vi "OpenExistingDataLogFile.vi"(6 "Chunk Read size, bytes":i32, 8 "error in (no error)":errorcluster, 9 "ExistingFilePath":path, 11 "ExistingFileMgr in":refnum<class "ExistingFileMgr.lvclass">) -> (0 "error out":errorcluster, 3 "ExistingFileMgr out":refnum<class "ExistingFileMgr.lvclass">)   [LabVIEW 2018, in "ExistingFileMgr.lvclass"]
uses:
  ExistingFileMgr.lvclass
  ExistingFileMgr.lvclass/ExistingFileMgr.ctl
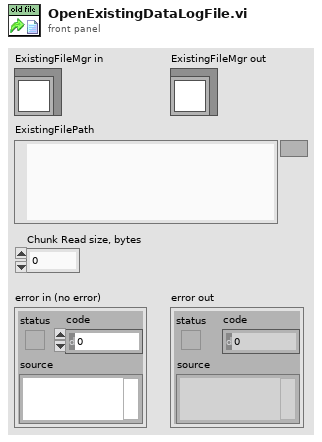
[diagram p1: front panel]
types:
  T1 = enum16{"open", "replace", "create", "open or create", "replace or create", "replace or create with confirmation"}
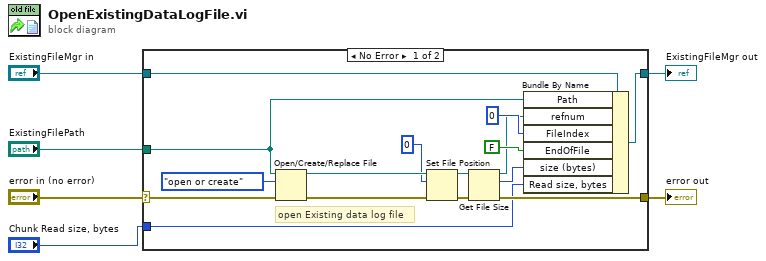
[diagram p0: block diagram]
diagram:
  n1 = case shown="No Error" "error in (no error)" {
    selector: "error in (no error)" -> [w16 w24]
    tunnel: [w8 w24] -> w2
    tunnel: [w20 w23] -> w3
    tunnel: "ExistingFileMgr in" -> [w21 w23]
    tunnel: "ExistingFilePath" -> [w17 _]
    tunnel: "Chunk Read size, bytes" -> [w7 _]
    frame No Error {
      # "open Existing data log file"
      n2 = Open/Create/Replace File(file path (use dialog)=w17, error in=w16, operation (0:open)=T1."open or create") -> (refnum out=w18:refnum<file>, error out=w19:errorcluster)  [unwired: 3 in, 1 out]
      n3 = Set File Position(offset (in bytes) (0)=i64 0, refnum=w18, error in=w19) -> (refnum out=w12:refnum<file>, error out=w9:errorcluster)  [unwired: 1 in]
      n4 = Get File Size(file=w12, error in=w9) -> (refnum out=w11:refnum<file>, size (in bytes)=w10:i64, 0:w8:errorcluster)
      n5 = Bundle By Name(cluster=w21, "Path"=w17, "refnum"=w11, "FileIndex"=i64 0, "EndOfFile"=FALSE, "size (bytes)"=w10, "Read size, bytes"=w7) -> (w20:refnum<class "ExistingFileMgr.lvclass">)
    }
    frame Error {
    }
  }
  "error out" <- w2
  "ExistingFileMgr out" <- w3
